vi "Pneumatiktest.vi"(8 "error in (no error)":errorcluster caption="Fehler (Eingang, kein Fehler)", 11 "Device ID":T1(ring)) -> (0 "error out":errorcluster caption="Fehler (Ausgang)", 3 "Device ID Out":T1(ring))   [LabVIEW 2010]
panel:
  out "leuft":u8(slide) scale=0.0..17.0
  in  "demo":bool
  in  "mitte":bool
  in  "ende":bool
  in  "rechts":bool
  in  "links":bool
  in  "vorne":bool
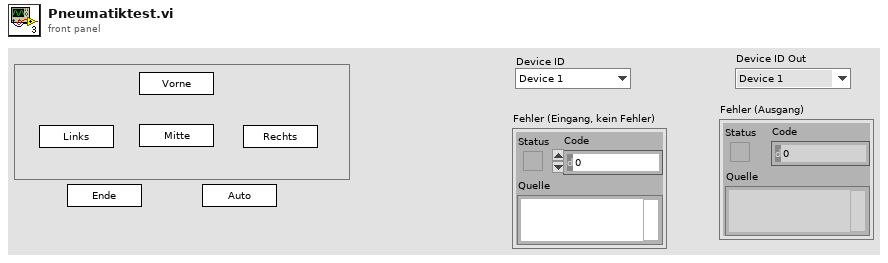
[diagram p1: front panel]
types:
  T1 = enum16{"Device 1", "Device 2", "Device 3", "Device 4", "Device 5", "Device 6", "Device 7", "Device 8"}
  T2 = enum8{"Power 1", "Power 2", "Power 3", "Power 4", "Power 5", "Power 6", "Power 7", "Power 8"}
  T3 = enum8{"Output 1 (O1)", "Output 2 (O2)", "Output 3 (O3)", "Output 4 (O4)", "Output 5 (O5)", "Output 6 (O6)", "Output 7 (O7)", "Output 8 (O8)"}
  T4 = enum8{"Robo Interface", "Extension 1", "Extension 2", "Extension 3"}
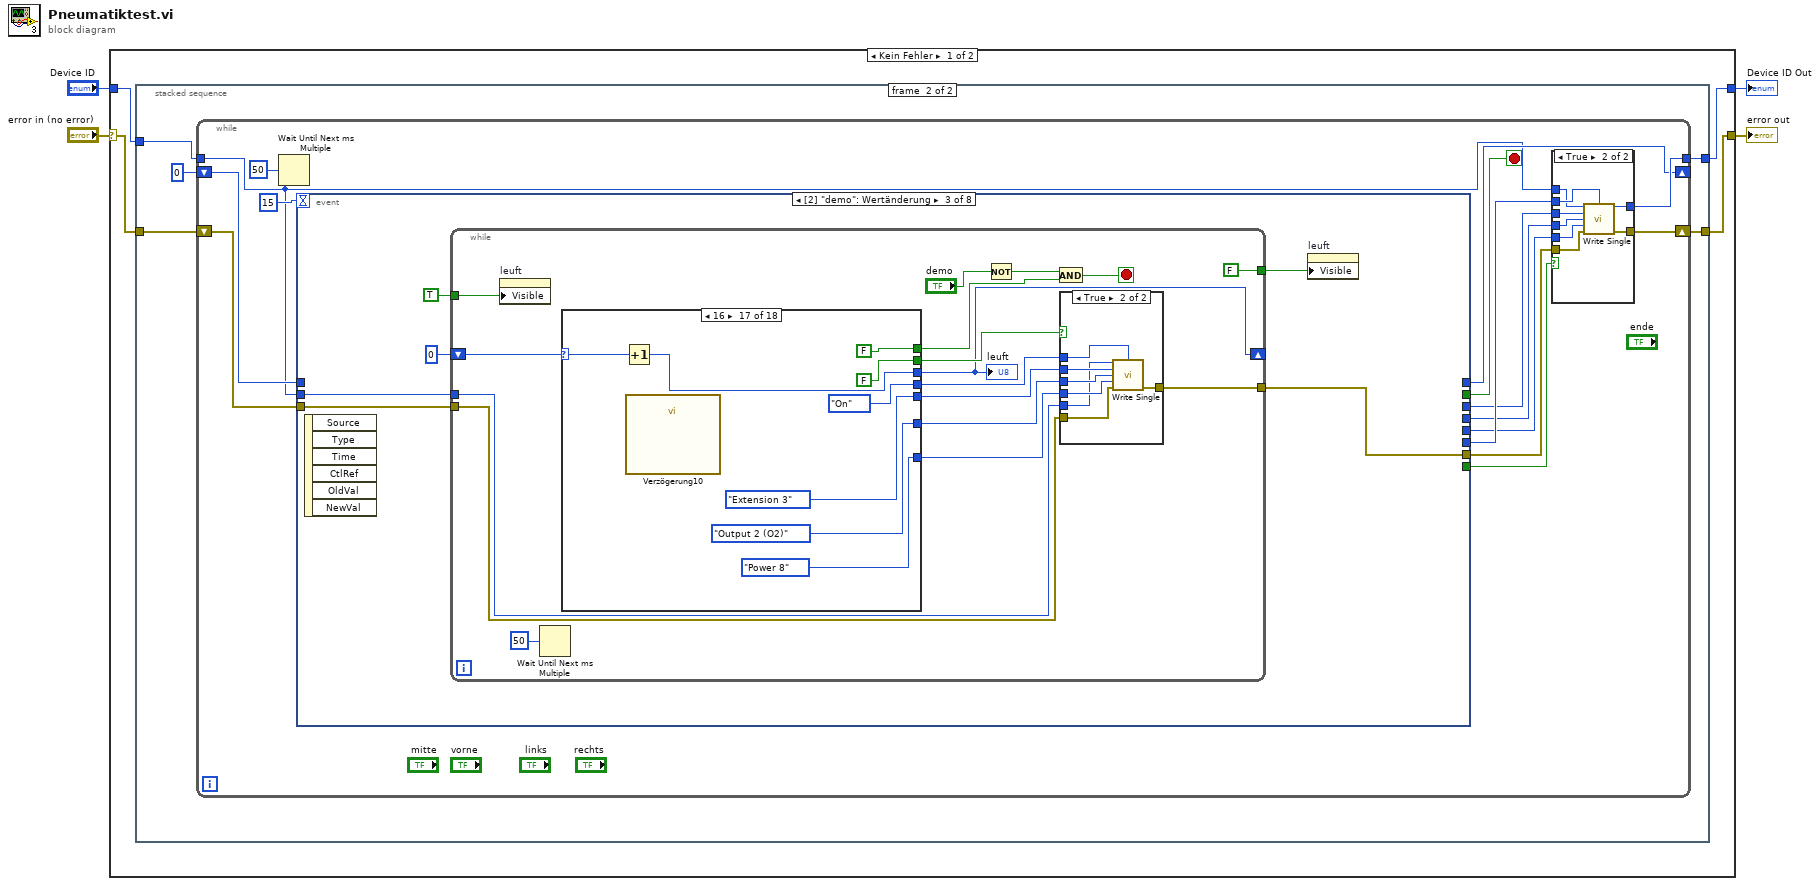
[diagram p0: block diagram]
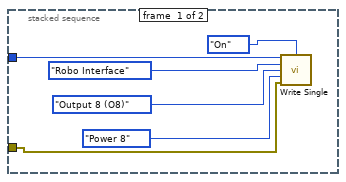
[diagram p2: hidden frame]
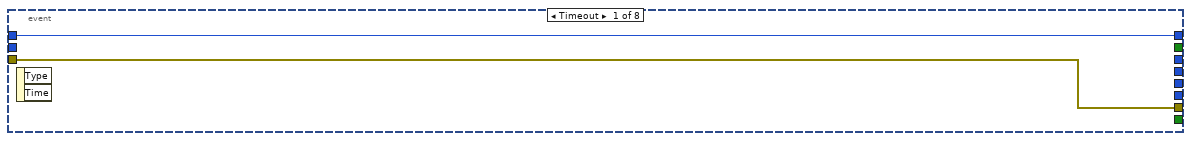
[diagram p3: hidden frame]
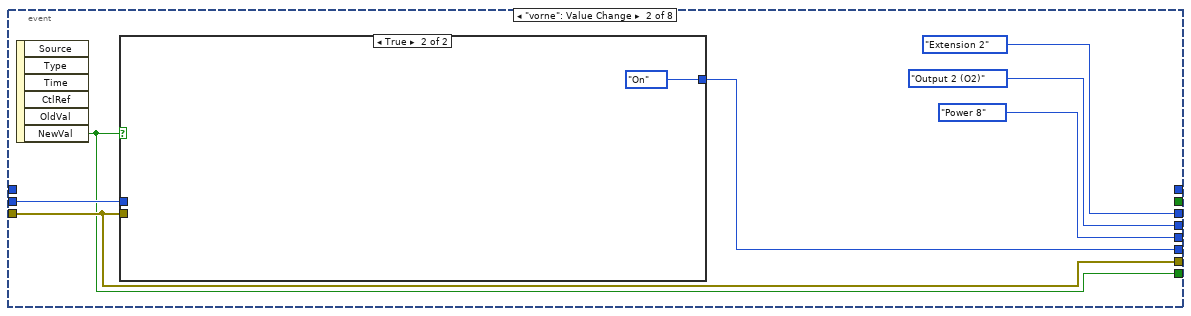
[diagram p4: hidden frame]
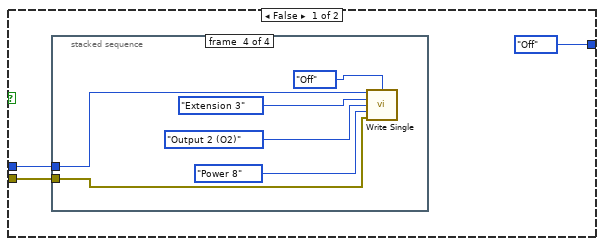
[diagram p5: hidden frame]
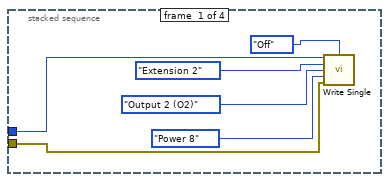
[diagram p6: hidden frame]
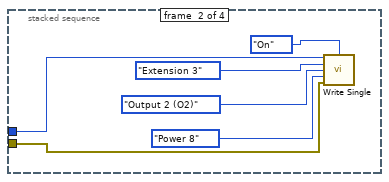
[diagram p7: hidden frame]
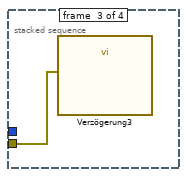
[diagram p8: hidden frame]
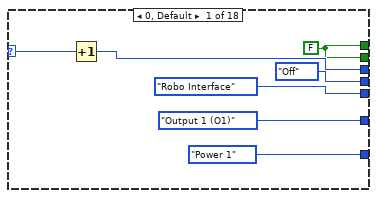
[diagram p9: hidden frame]
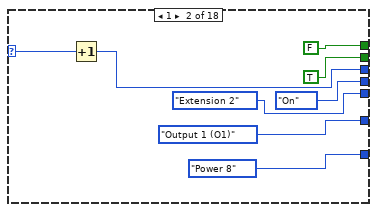
[diagram p10: hidden frame]
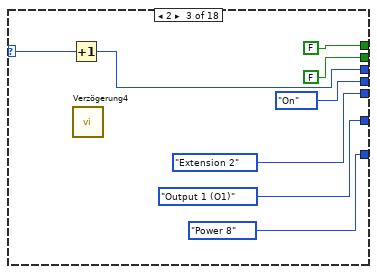
[diagram p11: hidden frame]
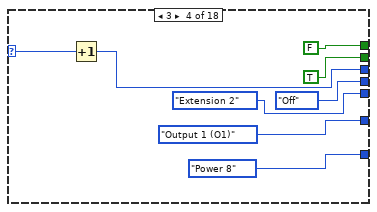
[diagram p12: hidden frame]
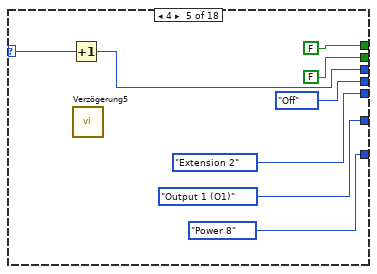
[diagram p13: hidden frame]
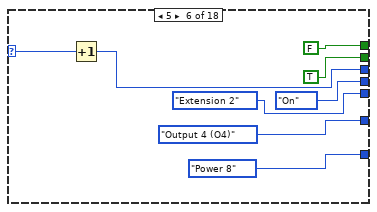
[diagram p14: hidden frame]
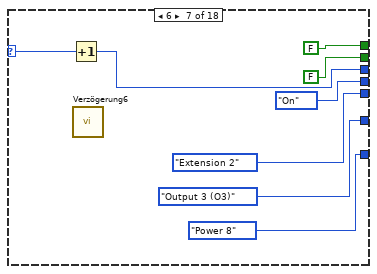
[diagram p15: hidden frame]
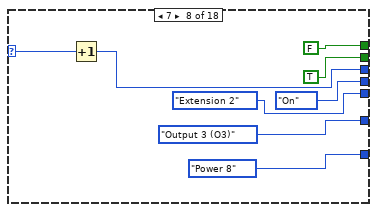
[diagram p16: hidden frame]
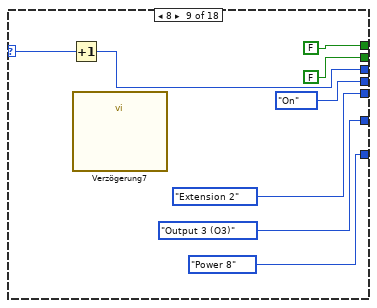
[diagram p17: hidden frame]
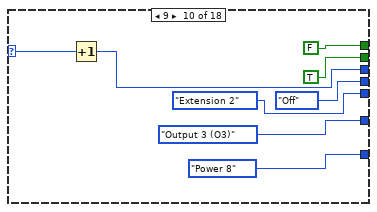
[diagram p18: hidden frame]
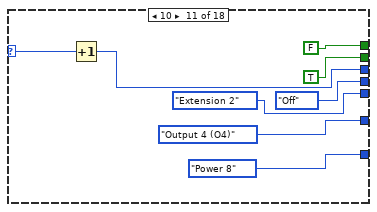
[diagram p19: hidden frame]
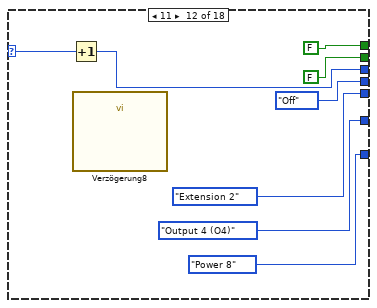
[diagram p20: hidden frame]
diagram:
  n1 = case shown="Kein Fehler" "error in (no error)" {
    selector: "error in (no error)" -> [w5 w328]
    tunnel: [w8 w328] -> w3
    tunnel: "Device ID" -> [w7 w327]
    tunnel: [w6 w327] -> w1
    frame No Error {
      n2 = stacked-sequence {
        tunnel: [_ w19] -> w8
        tunnel: w7 -> [w14 w18]
        tunnel: [_ w17] -> w6
        tunnel: w5 -> [w9 w16]
        frame #0 {
          n3 = call "Write Single.vi"("Device ID"=w14, "Output_Action"=enum8{"Off", "On"}."On", "Module"=T4."Robo Interface", "Single_Output"=T3."Output 8 (O8)", "Output_PWM"=T2."Power 8", "error in"=w9) -> ()  [unwired: 10 out]
        }
        frame #1 {
          n4 = while {
            shift-right: [w27] -> w19
            shift-left: w16 -> [w26]
            tunnel: w18 -> [w20]
            tunnel: [w25] -> w17
            shift-right: [w21] -> _
            shift-left: 0 -> [w22]
            stop <- w24 stop-if-true
            n5 = Wait Until Next ms Multiple(millisecond multiple=50) -> ()  [unwired: 1 out]
            n6 = event shown="[2] \"demo\": Wertänderung" {
              selector: _ -> [_ _ _ _ _ _ _ _]
              dyn-events: _ -> [_ _ _ _ _ _ _ _]
              timeout: 15 -> [_ _ _ _ _ _ _ _]
              tunnel: [_ w37 _ TRUE TRUE TRUE TRUE TRUE] -> w33
              tunnel: [_ w40 _ w243 w251 w259 enum8{"Off", "On"}."Off" ("Output_Action") enum8{"Off", "On"}."Off" ("Output_Action")] -> w32
              tunnel: [_ T4."Extension 2" ("Module") _ T4."Extension 2" ("Module") T4."Extension 2" ("Module") T4."Extension 2" ("Module") T4."Robo Interface" ("Module") T4."Robo Interface" ("Module")] -> w31
              tunnel: [_ T3."Output 2 (O2)" ("Single_Output") _ T3."Output 1 (O1)" ("Single_Output") T3."Output 4 (O4)" ("Single_Output") T3."Output 3 (O3)" ("Single_Output") T3."Output 8 (O8)" ("Single_Output") T3."Output 8 (O8)" ("Single_Output")] -> w30
              tunnel: [_ T2."Power 8" ("Output_PWM") _ T2."Power 8" ("Output_PWM") T2."Power 8" ("Output_PWM") T2."Power 8" ("Output_PWM") _ _] -> w29
              tunnel: [w36 w38 w71 _ _ _ _ _] -> w28
              tunnel: w26 -> [w36 w38 w72 _ _ _ w265 w292]
              tunnel: [_ _ _ _ _ _ TRUE TRUE] -> w24
              tunnel: w22 -> [w35 _ _ _ _ _ _ _]
              tunnel: w20 -> [_ w39 w69 _ _ _ w266 w293]
              tunnel: [w35 _ _ _ _ _ _ _] -> w21
              event Timeout {
                n7 = event-data() -> ()  [unwired: 3 out]
              }
              event "vorne": Value Change {
                n8 = event-data() -> ("NewVal"=w37:bool)  [unwired: 6 out]
                n9 = case shown="TRUE" w37 {
                  tunnel: [enum8{"Off", "On"}."Off" ("Output_Action") enum8{"Off", "On"}."On" ("Output_Action")] -> w40
                  tunnel: w39 -> [w45 _]
                  tunnel: w38 -> [w44 _]
                  frame False {
                    n10 = stacked-sequence {
                      tunnel: w45 -> [w47 w58 _ w62]
                      tunnel: w44 -> [w48 w53 w59 w60]
                      frame #0 {
                        n11 = call "Write Single.vi"("Device ID"=w47, "Output_Action"=enum8{"Off", "On"}."Off", "Module"=T4."Extension 2", "Single_Output"=T3."Output 2 (O2)", "Output_PWM"=T2."Power 8", "error in"=w48) -> ()  [unwired: 10 out]
                      }
                      frame #1 {
                        n12 = call "Write Single.vi"("Device ID"=w58, "Output_Action"=enum8{"Off", "On"}."On", "Module"=T4."Extension 3", "Single_Output"=T3."Output 2 (O2)", "Output_PWM"=T2."Power 8", "error in"=w53) -> ()  [unwired: 10 out]
                      }
                      frame #2 {
                        n13 = call "Verzögerung3"("error in (no error)"=w59) -> ()  [unwired: 1 in, 10 out]
                      }
                      frame #3 {
                        n14 = call "Write Single.vi"("Device ID"=w62, "Output_Action"=enum8{"Off", "On"}."Off", "Module"=T4."Extension 3", "Single_Output"=T3."Output 2 (O2)", "Output_PWM"=T2."Power 8", "error in"=w60) -> ()  [unwired: 10 out]
                      }
                    }
                  }
                  frame True {
                  }
                }
              }
              event "demo": Value Change {
                n15 = event-data() -> ()  [unwired: 7 out]
                n16 = while {
                  tunnel: w72 -> [w85]
                  tunnel: [w84] -> w71
                  shift-right: [w73] -> _
                  shift-left: 0 -> [w81]
                  tunnel: w69 -> [w77]
                  tunnel: TRUE -> [w75]
                  tunnel: [FALSE] -> w67
                  stop <- w79 stop-if-true
                  n17 = property on="leuft" class="Schieber (strikt)"("Visible"=w75) -> ()  [unwired: 2 in, 2 out]
                  n18 = Wait Until Next ms Multiple(millisecond multiple=50) -> ()  [unwired: 1 out]
                  n19 = case shown="16" w81 {
                    selector: w81 -> [w92 w100 w108 w116 w124 w132 w140 w148 w156 w164 w172 w180 w188 w196 w202 w210 w218 _]
                    tunnel: [T4."Robo Interface" ("Module") T4."Extension 2" ("Module") T4."Extension 2" ("Module") T4."Extension 2" ("Module") T4."Extension 2" ("Module") T4."Extension 2" ("Module") T4."Extension 2" ("Module") T4."Extension 2" ("Module") T4."Extension 2" ("Module") T4."Extension 2" ("Module") T4."Extension 2" ("Module") T4."Extension 2" ("Module") T4."Extension 2" ("Module") T4."Extension 2" ("Module") T4."Extension 2" ("Module") T4."Extension 3" ("Module") T4."Extension 3" ("Module") T4."Extension 3" ("Module")] -> w89
                    tunnel: [T3."Output 1 (O1)" ("Single_Output") T3."Output 1 (O1)" ("Single_Output") T3."Output 1 (O1)" ("Single_Output") T3."Output 1 (O1)" ("Single_Output") T3."Output 1 (O1)" ("Single_Output") T3."Output 4 (O4)" ("Single_Output") T3."Output 3 (O3)" ("Single_Output") T3."Output 3 (O3)" ("Single_Output") T3."Output 3 (O3)" ("Single_Output") T3."Output 3 (O3)" ("Single_Output") T3."Output 4 (O4)" ("Single_Output") T3."Output 4 (O4)" ("Single_Output") T3."Output 2 (O2)" ("Single_Output") T3."Output 2 (O2)" ("Single_Output") T3."Output 2 (O2)" ("Single_Output") T3."Output 2 (O2)" ("Single_Output") T3."Output 2 (O2)" ("Single_Output") T3."Output 2 (O2)" ("Single_Output")] -> w88
                    tunnel: [T2."Power 1" ("Output_PWM") T2."Power 8" ("Output_PWM") T2."Power 8" ("Output_PWM") T2."Power 8" ("Output_PWM") T2."Power 8" ("Output_PWM") T2."Power 8" ("Output_PWM") T2."Power 8" ("Output_PWM") T2."Power 8" ("Output_PWM") T2."Power 8" ("Output_PWM") T2."Power 8" ("Output_PWM") T2."Power 8" ("Output_PWM") T2."Power 8" ("Output_PWM") T2."Power 8" ("Output_PWM") T2."Power 8" ("Output_PWM") T2."Power 8" ("Output_PWM") T2."Power 8" ("Output_PWM") T2."Power 8" ("Output_PWM") T2."Power 8" ("Output_PWM")] -> w87
                    tunnel: [enum8{"Off", "On"}."Off" ("Output_Action") enum8{"Off", "On"}."On" ("Output_Action") enum8{"Off", "On"}."On" ("Output_Action") enum8{"Off", "On"}."Off" ("Output_Action") enum8{"Off", "On"}."Off" ("Output_Action") enum8{"Off", "On"}."On" ("Output_Action") enum8{"Off", "On"}."On" ("Output_Action") enum8{"Off", "On"}."On" ("Output_Action") enum8{"Off", "On"}."On" ("Output_Action") enum8{"Off", "On"}."Off" ("Output_Action") enum8{"Off", "On"}."Off" ("Output_Action") enum8{"Off", "On"}."Off" ("Output_Action") enum8{"Off", "On"}."On" ("Output_Action") enum8{"Off", "On"}."On" ("Output_Action") enum8{"Off", "On"}."Off" ("Output_Action") enum8{"Off", "On"}."On" ("Output_Action") enum8{"Off", "On"}."On" ("Output_Action") enum8{"Off", "On"}."Off" ("Output_Action")] -> w86
                    tunnel: [w90 TRUE FALSE TRUE FALSE TRUE FALSE TRUE FALSE TRUE TRUE FALSE TRUE FALSE TRUE TRUE FALSE TRUE] -> w82
                    tunnel: [w91 w99 w107 w115 w123 w131 w139 w147 w155 w163 w171 w179 w187 w195 w201 w209 w217 0] -> w73
                    tunnel: [w90 FALSE FALSE FALSE FALSE FALSE FALSE FALSE FALSE FALSE FALSE FALSE FALSE FALSE FALSE FALSE FALSE TRUE] -> w78
                    frame 0, Default {
                      w90 = FALSE
                      n20 = Increment(x=w92) -> (x+1=w91:i32)
                    }
                    frame 1 {
                      n21 = Increment(x=w100) -> (x+1=w99:i32)
                    }
                    frame 2 {
                      n22 = Increment(x=w108) -> (x+1=w107:i32)
                      n23 = call "Verzögerung4"() -> ()  [unwired: 2 in, 10 out]
                    }
                    frame 3 {
                      n24 = Increment(x=w116) -> (x+1=w115:i32)
                    }
                    frame 4 {
                      n25 = Increment(x=w124) -> (x+1=w123:i32)
                      n26 = call "Verzögerung5"() -> ()  [unwired: 2 in, 10 out]
                    }
                    frame 5 {
                      n27 = Increment(x=w132) -> (x+1=w131:i32)
                    }
                    frame 6 {
                      n28 = Increment(x=w140) -> (x+1=w139:i32)
                      n29 = call "Verzögerung6"() -> ()  [unwired: 2 in, 10 out]
                    }
                    frame 7 {
                      n30 = Increment(x=w148) -> (x+1=w147:i32)
                    }
                    frame 8 {
                      n31 = Increment(x=w156) -> (x+1=w155:i32)
                      n32 = call "Verzögerung7"() -> ()  [unwired: 2 in, 10 out]
                    }
                    frame 9 {
                      n33 = Increment(x=w164) -> (x+1=w163:i32)
                    }
                    frame 10 {
                      n34 = Increment(x=w172) -> (x+1=w171:i32)
                    }
                    frame 11 {
                      n35 = Increment(x=w180) -> (x+1=w179:i32)
                      n36 = call "Verzögerung8"() -> ()  [unwired: 2 in, 10 out]
                    }
                    frame 12 {
                      n37 = Increment(x=w188) -> (x+1=w187:i32)
                    }
                    frame 13 {
                      n38 = Increment(x=w196) -> (x+1=w195:i32)
                      n39 = call "Verzögerung9"() -> ()  [unwired: 2 in, 10 out]
                    }
                    frame 14 {
                      n40 = Increment(x=w202) -> (x+1=w201:i32)
                    }
                    frame 15 {
                      n41 = Increment(x=w210) -> (x+1=w209:i32)
                    }
                    frame 16 {
                      n42 = Increment(x=w218) -> (x+1=w217:i32)
                      n43 = call "Verzögerung10"() -> ()  [unwired: 2 in, 10 out]
                    }
                    frame 17 {
                    }
                  }
                  "leuft" <- w73
                  n44 = Not(x="demo") -> (.not. x?=w76:bool)
                  n45 = And(x=w76, y=w78) -> (x .and. y?=w79:bool)
                  n46 = case shown="True" w82 {
                    tunnel: w85 -> [w232 w239]
                    tunnel: [w232 w238] -> w84
                    tunnel: w89 -> [_ w237]
                    tunnel: w88 -> [_ w236]
                    tunnel: w87 -> [_ w235]
                    tunnel: w86 -> [_ w234]
                    tunnel: w77 -> [_ w233]
                    frame False {
                    }
                    frame True {
                      n47 = call "Write Single.vi"("Device ID"=w233, "Output_Action"=w234, "Module"=w237, "Single_Output"=w236, "Output_PWM"=w235, "error in"=w239) -> ("error out"=w238:errorcluster)  [unwired: 9 out]
                    }
                  }
                }
                n48 = property on="leuft" class="Schieber (strikt)"("Visible"=w67) -> ()  [unwired: 2 in, 2 out]
              }
              event "links": Value Change {
                n49 = event-data() -> ("NewVal"=w245:bool)  [unwired: 6 out]
                n50 = case shown="FALSE" w245 {
                  tunnel: [enum8{"Off", "On"}."Off" ("Output_Action") enum8{"Off", "On"}."On" ("Output_Action")] -> w243
                  frame False {
                  }
                  frame True {
                  }
                }
              }
              event "mitte": Value Change {
                n51 = event-data() -> ("NewVal"=w253:bool)  [unwired: 6 out]
                n52 = case shown="FALSE" w253 {
                  tunnel: [enum8{"Off", "On"}."Off" ("Output_Action") enum8{"Off", "On"}."On" ("Output_Action")] -> w251
                  frame False {
                  }
                  frame True {
                  }
                }
              }
              event "rechts": Value Change {
                n53 = event-data() -> ("NewVal"=w261:bool)  [unwired: 6 out]
                n54 = case shown="FALSE" w261 {
                  tunnel: [enum8{"Off", "On"}."Off" ("Output_Action") enum8{"Off", "On"}."On" ("Output_Action")] -> w259
                  frame False {
                  }
                  frame True {
                  }
                }
              }
              event "ende": Value Change {
                n55 = event-data() -> ()  [unwired: 2 out]
                n56 = stacked-sequence {
                  tunnel: w266 -> [w272 w278 _ w286]
                  tunnel: w265 -> [w271 w277 w283 w284]
                  frame #0 {
                    n57 = call "Write Single.vi"("Device ID"=w272, "Output_Action"=enum8{"Off", "On"}."Off", "Module"=T4."Robo Interface", "Single_Output"=T3."Output 8 (O8)", "Output_PWM"=T2."Power 8", "error in"=w271) -> ()  [unwired: 10 out]
                  }
                  frame #1 {
                    n58 = call "Write Single.vi"("Device ID"=w278, "Output_Action"=enum8{"Off", "On"}."On", "Module"=T4."Extension 3", "Single_Output"=T3."Output 1 (O1)", "Output_PWM"=T2."Power 8", "error in"=w277) -> ()  [unwired: 10 out]
                  }
                  frame #2 {
                    n59 = call "Verzögerung"("error in (no error)"=w283) -> ()  [unwired: 1 in, 10 out]
                  }
                  frame #3 {
                    n60 = call "Write Single.vi"("Device ID"=w286, "Output_Action"=enum8{"Off", "On"}."Off", "Module"=T4."Extension 3", "Single_Output"=T3."Output 1 (O1)", "Output_PWM"=T2."Power 8", "error in"=w284) -> ()  [unwired: 10 out]
                  }
                }
              }
              event Panel Close? {
                n61 = event-data() -> ()  [unwired: 2 out]
                n62 = stacked-sequence {
                  tunnel: w293 -> [w299 w305 _ w313]
                  tunnel: w292 -> [w298 w304 w310 w311]
                  frame #0 {
                    n63 = call "Write Single.vi"("Device ID"=w299, "Output_Action"=enum8{"Off", "On"}."Off", "Module"=T4."Robo Interface", "Single_Output"=T3."Output 8 (O8)", "Output_PWM"=T2."Power 8", "error in"=w298) -> ()  [unwired: 10 out]
                  }
                  frame #1 {
                    n64 = call "Write Single.vi"("Device ID"=w305, "Output_Action"=enum8{"Off", "On"}."On", "Module"=T4."Extension 3", "Single_Output"=T3."Output 1 (O1)", "Output_PWM"=T2."Power 8", "error in"=w304) -> ()  [unwired: 10 out]
                  }
                  frame #2 {
                    n65 = call "Verzögerung2"("error in (no error)"=w310) -> ()  [unwired: 1 in, 10 out]
                  }
                  frame #3 {
                    n66 = call "Write Single.vi"("Device ID"=w313, "Output_Action"=enum8{"Off", "On"}."Off", "Module"=T4."Extension 3", "Single_Output"=T3."Output 1 (O1)", "Output_PWM"=T2."Power 8", "error in"=w311) -> ()  [unwired: 10 out]
                  }
                }
                n67 = event-data("Discard?"=TRUE ("Verwerfen?")) -> ()  [unwired: 1 in, 1 out]
              }
            }
            n68 = case shown="True" w33 {
              tunnel: w28 -> [w318 w326]
              tunnel: [w318 w325] -> w27
              tunnel: w31 -> [_ w324]
              tunnel: w30 -> [_ w323]
              tunnel: w29 -> [_ w322]
              tunnel: w32 -> [_ w321]
              tunnel: [w317 w320] -> w25
              tunnel: w20 -> [w317 w319]
              frame False {
              }
              frame True {
                n69 = call "Write Single.vi"("Device ID"=w319, "Output_Action"=w321, "Module"=w324, "Single_Output"=w323, "Output_PWM"=w322, "error in"=w326) -> ("Device ID Out"=w320:T1, "error out"=w325:errorcluster)  [unwired: 8 out]
              }
            }
          }
        }
      }
    }
    frame Error {
    }
  }
  "error out" <- w3
  "Device ID Out" <- w1
